vi "Example.vi"() -> ()   [LabVIEW 2018, in "Markdown.lvlib"]
doc: "Open and run the `Example.vi` to see an how to export a LabVIEW Library (*.lvlib) to markdown documentation.\n\nThis is useful to auto-generate API help documentation for GitHub."
uses:
  Markdown.lvlib
panel:
  out "Images":path[](array[path])
  out "Markdown out":path
  out "error out":errorcluster
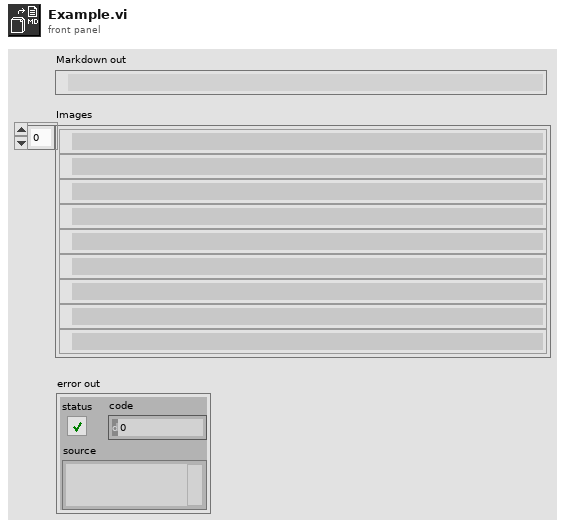
[diagram p1: front panel]
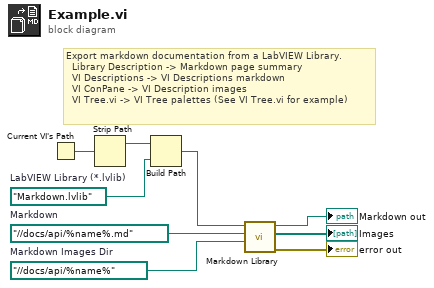
[diagram p0: block diagram]
diagram:
  w1 = path "../../docs/api/%name%"  # Markdown Images Dir
  w2 = path "../../docs/api/%name%.md"  # Markdown
  w7 = path "Markdown.lvlib"  # LabVIEW Library (*.lvlib)
  # "Export markdown documentation from a LabVIEW Library.\n  Library Description -> Markdown page summary\n  VI Descriptions -> VI Descriptions markdown\n  VI ConPane -> VI Description images\n  VI Tree.vi -> VI Tree palettes (See VI Tree.vi for example)"
  n1 = Current VI's Path() -> (path=w9:path)
  n2 = Strip Path(path=w9) -> (stripped path=w8:path)  [unwired: 1 out]
  n3 = Build Path(base path=w8, name or relative path=w7) -> (appended path=w6:path)
  n4 = call "Markdown Library.vi"("Markdown Images Dir (..\\..\\docs\\%name%)"=w1, "Markdown in (..\\..\\docs\\%name%.md)"=w2, "Library Path (*.lvlib)"=w6) -> ("error out"=→"error out":errorcluster, "Images"=→"Images":path[], "Markdown out"=→"Markdown out":path)  [unwired: 6 in]
